vi "Discovery Client Enumerate Services.vi"(5 "Request Data":T1={"provided_interface"="UnitTestProvidedInterface"}, 11 "error in (no error)":errorcluster) -> (6 "Response Data":T2, 15 "error out":errorcluster)   [LabVIEW 2020]
uses:
  Discovery Client_lv/Discovery_client/RPC Messages/ni_measurementlink_discovery_v1_EnumerateServicesResponse.ctl
  Discovery Client_lv/Discovery_client/RPC Messages/ni_measurementlink_discovery_v1_ServiceDescriptor.ctl
  Discovery Client_lv/Discovery_client/RPC Messages/ni_measurementlink_discovery_v1_EnumerateServicesRequest.ctl
  Discovery Client_lv/Discovery_client/Discovery_client.lvlib
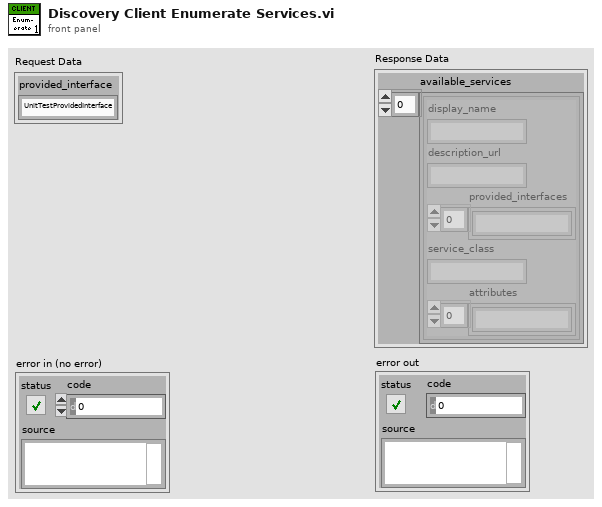
[diagram p1: front panel]
types:
  T1 = typedef "Discovery_client.lvlib/ni_measurementlink_discovery_v1_EnumerateServicesRequest.ctl" = cluster{"provided_interface":string}
  T2 = typedef "Discovery_client.lvlib/ni_measurementlink_discovery_v1_EnumerateServicesResponse.ctl" = cluster{"available_services":T3[]}
  T3 = typedef "Discovery_client.lvlib/ni_measurementlink_discovery_v1_ServiceDescriptor.ctl" = cluster{"display_name":string, "description_url":string, "provided_interfaces":string[], "service_class":string, "attributes":string[]}
  T4 = typedef "grpc-lvsupport-release.lvlib/grpcId.ctl" = u64
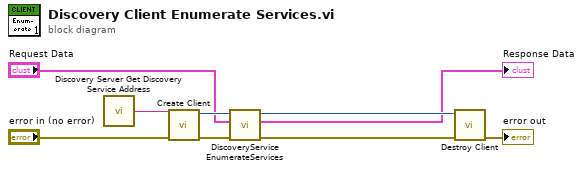
[diagram p0: block diagram]
diagram:
  n1 = call "Discovery Server Get Discovery Service Address.vi"() -> ("address"=w9:string)  [unwired: 15 in]
  n2 = call "Create Client.vi"("error in"="error in (no error)", "address"=w9) -> ("error out"=w8:errorcluster, "gRPC ID Out"=w6:T4)  [unwired: 8 in]
  n3 = call "DiscoveryService EnumerateServices.vi"("error in"=w8, "Request Data"="Request Data", "gRPC ID"=w6) -> ("error out"=w7:errorcluster, "Response Data"=→"Response Data":T2, "gRPC ID out"=w5:T4)  [unwired: 6 in]
  n4 = call "Destroy Client.vi"("error in"=w7, "gRPC ID"=w5) -> ("error out"=→"error out":errorcluster)  [unwired: 9 in]
